vi "Continuous Graph Update.vi"(0 "SequenceContext":refnum<k7>, 2 "Stop_V":dbl) -> (4 "Stop Button Out":bool)   [LabVIEW 2013]
uses:
  <vilib>/addons/TestStand/_TSUtility.llb/TestStand - Get Property Value (Numeric Array).vi
panel:
  out "Graph Cluster":T1
  in  "Stop Button":bool
  in  "error in (no error)":errorcluster
  out "Error Out":errorcluster
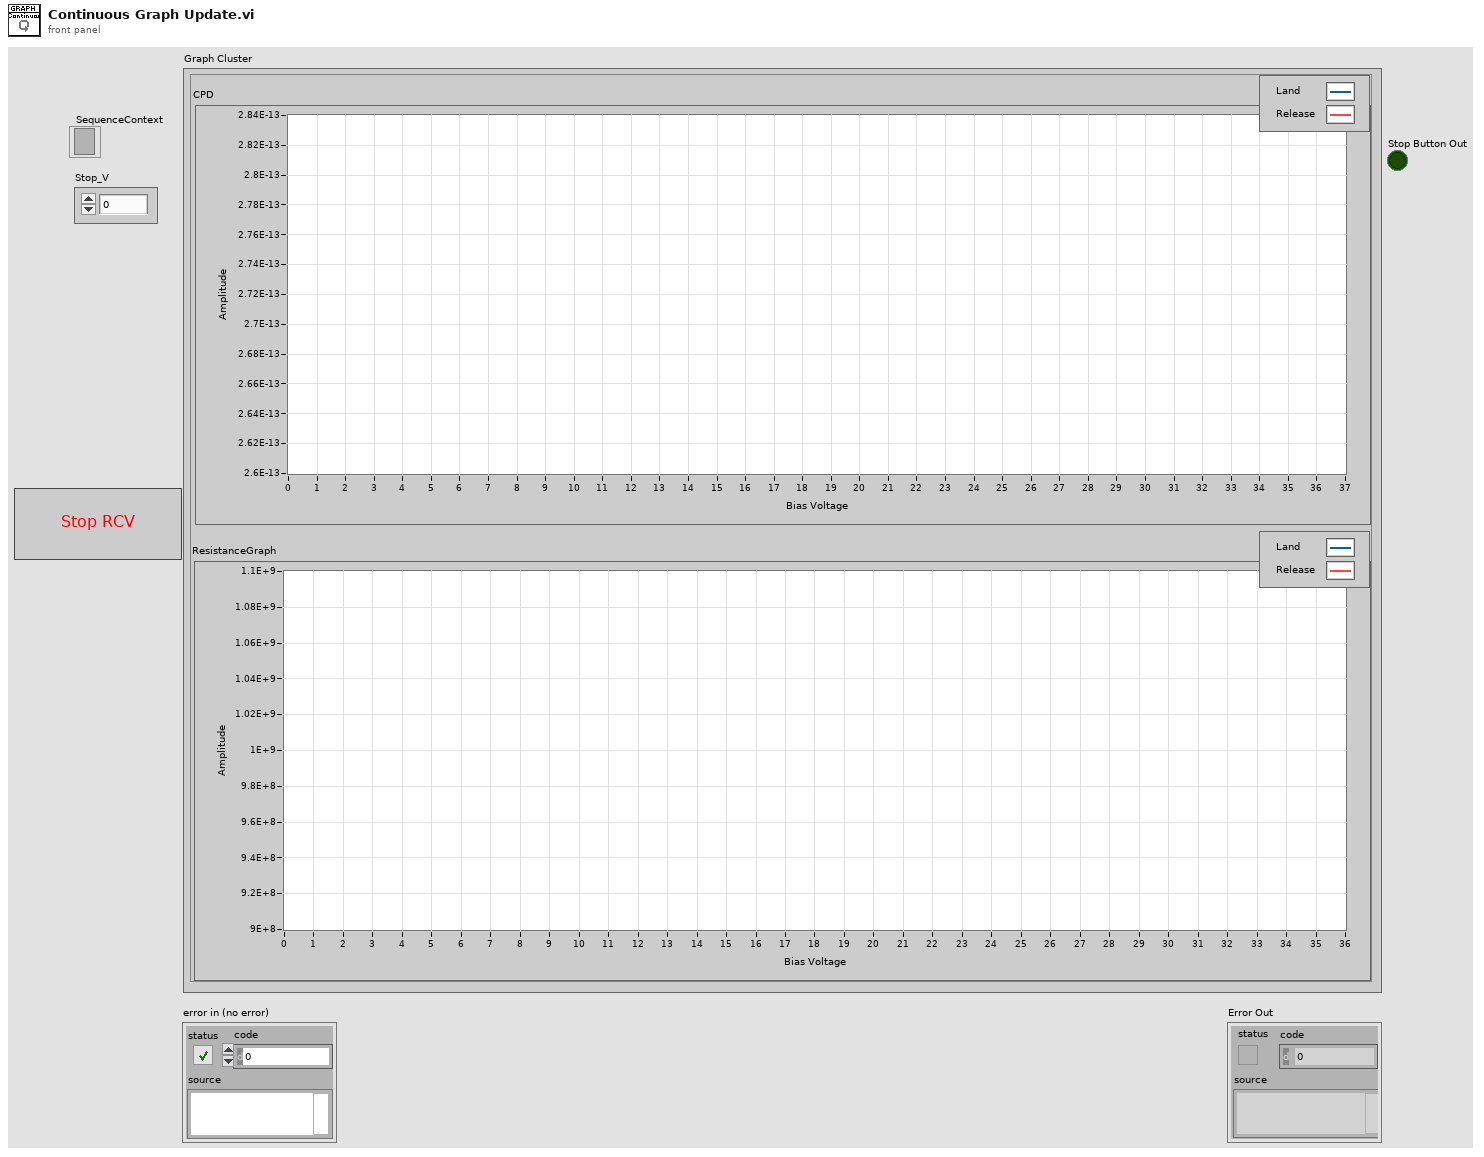
[diagram p1: front panel]
types:
  T1 = cluster{"ResistanceGraph":cluster{dbl[], dbl[]}[], "CPD":cluster{dbl[], dbl[]}[]}
  T2 = typedef "TestStand - Status Monitor.ctl" = cluster{"Sequence Context":refnum<k7>, "Execution":refnum<k7>, "Termination Monitor":refnum<k7>}
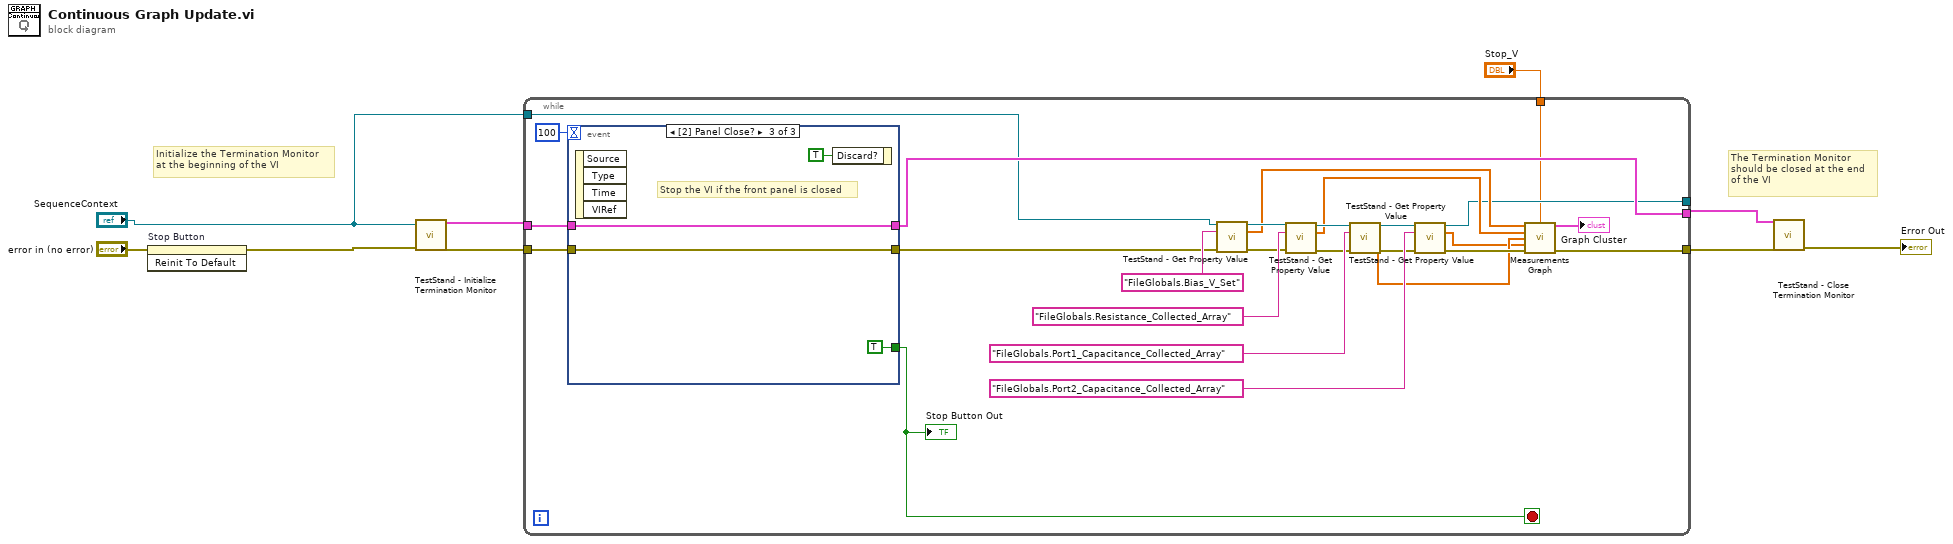
[diagram p0: block diagram]
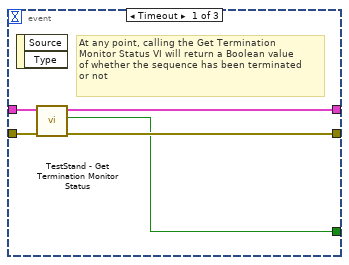
[diagram p2: hidden frame]
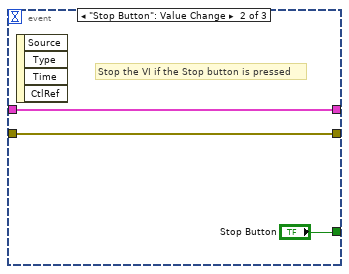
[diagram p3: hidden frame]
diagram:
  # "Initialize the Termination Monitor\nat the beginning of the VI"
  # "The Termination Monitor\nshould be closed at the end\nof the VI"
  n1 = invoke on="Stop Button" class="Bool (strict)" method="Reinit To Default"(error in="error in (no error)") -> (error out=w4:errorcluster)  [unwired: 2 in, 2 out]
  n2 = call <vilib>:"TestStand - Initialize Termination Monitor.vi"("error in (no error)"=w4, "Sequence Context In"="SequenceContext") -> ("error out"=w8:errorcluster, "Status Monitor Out"=w9:T2)  [unwired: 8 in]
  n3 = while {
    tunnel: w8 -> [w33]
    tunnel: [w35] -> w7
    tunnel: w9 -> [w30]
    tunnel: [w31] -> w6
    tunnel: "SequenceContext" -> [w17]
    tunnel: [w11] -> _
    tunnel: "Stop_V" -> [w10]
    stop <- w32 stop-if-true
    n4 = event shown="[2] Panel Close?" {
      selector: _ -> [_ _ _]
      dyn-events: _ -> [_ _ _]
      timeout: 100 -> [_ _ _]
      tunnel: w30 -> [w36 w41 w44]
      tunnel: w33 -> [w40 w42 w46]
      tunnel: [w39 w42 w46] -> w19
      tunnel: [w38 w41 w44] -> w31
      tunnel: [w37 "Stop Button" TRUE ("Stop Button")] -> w32
      event Timeout {
        # "At any point, calling the Get Termination\nMonitor Status VI will return a Boolean value\nof whether the sequence has been terminated \nor not"
        n5 = event-data() -> ()  [unwired: 1 in, 2 out]
        n6 = call <vilib>:"TestStand - Get Termination Monitor Status.vi"("error in (no error)"=w40, "Status Monitor In"=w36) -> ("error out"=w39:errorcluster, "Terminating or Aborting"=w37:bool, "Status Monitor Out"=w38:T2)  [unwired: 7 in]
      }
      event "Stop Button": Value Change {
        # "Stop the VI if the Stop button is pressed"
        n7 = event-data() -> ()  [unwired: 1 in, 4 out]
      }
      event Panel Close? {
        # "Stop the VI if the front panel is closed"
        n8 = event-data() -> ()  [unwired: 1 in, 4 out]
        n9 = event-data("Discard?"=TRUE) -> ()  [unwired: 1 in, 1 out]
      }
    }
    "Stop Button Out" <- w32
    n10 = call-poly <vilib>:"TestStand - Get Property Value.vi"("Sequence Context In"=w17, "Lookup String"="FileGlobals.Bias_V_Set", "error in (no error)"=w19) -> ("Sequence Context Out"=w27:refnum<k7>, "Value"=w16:dbl[], "error out"=w20:errorcluster)  [unwired: 10 out]
    n11 = call-poly <vilib>:"TestStand - Get Property Value.vi"("Sequence Context In"=w27, "Lookup String"="FileGlobals.Resistance_Collected_Array", "error in (no error)"=w20) -> ("Sequence Context Out"=w28:refnum<k7>, "Value"=w15:dbl[], "error out"=w21:errorcluster)  [unwired: 10 out]
    n12 = call-poly <vilib>:"TestStand - Get Property Value.vi"("Sequence Context In"=w28, "Lookup String"="FileGlobals.Port1_Capacitance_Collected_Array", "error in (no error)"=w21) -> ("Sequence Context Out"=w26:refnum<k7>, "Value"=w14:dbl[], "error out"=w22:errorcluster)  [unwired: 10 out]
    n13 = call-poly <vilib>:"TestStand - Get Property Value.vi"("Sequence Context In"=w26, "Lookup String"="FileGlobals.Port2_Capacitance_Collected_Array", "error in (no error)"=w22) -> ("Sequence Context Out"=w11:refnum<k7>, "Value"=w13:dbl[], "error out"=w18:errorcluster)  [unwired: 10 out]
    n14 = call "Measurements Graph.vi"("Bias Voltage"=w16, "Stop_V"=w10, "Resitance"=w15, "Port 1 Cap"=w14, "Port 2 Cap"=w13, "Error In"=w18) -> ("Graph Cluster"=→"Graph Cluster":T1, "Error Out"=w35:errorcluster)  [unwired: 8 in]
  }
  n15 = call <vilib>:"TestStand - Close Termination Monitor.vi"("error in (no error)"=w7, "Status Monitor In"=w6) -> ("error out"=→"Error Out":errorcluster)  [unwired: 9 in]
